vi "TestTCP.vi"() -> ()   [LabVIEW 2011]
panel:
  out "Boolean":bool
  out "Error Out":errorcluster
  out "data out":string
  in  "port":u16=9000
  in  "Stop Button":bool
  out "NaN/Path/Refnum?":bool
  in  "TCP Network Connection Refnum":refnum<k5>
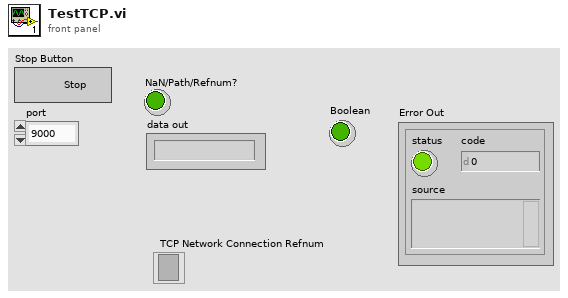
[diagram p1: front panel]
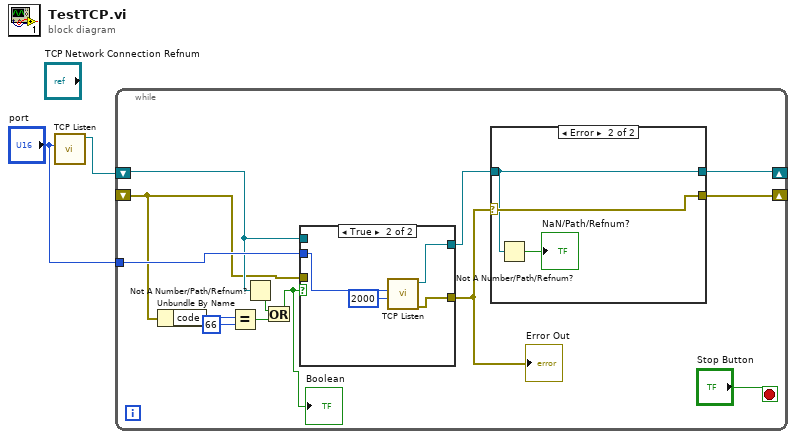
[diagram p0: block diagram]
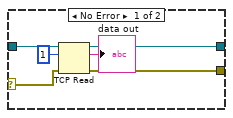
[diagram p3: hidden frame]
diagram:
  n1 = call <vilib>:"TCP Listen.vi"("port"="port") -> ("connection ID"=w2:refnum<k5>)  [unwired: 6 in, 4 out]
  n2 = while {
    shift-right: [w15] -> _
    shift-left: _ -> [w6]
    shift-right: [w14] -> _
    shift-left: w2 -> [w7]
    tunnel: "port" -> [w12]
    stop <- "Stop Button" stop-if-true
    n3 = Unbundle By Name(w6) -> ("code"=w9:i32)
    n4 = Equal?(x=w9, y=66) -> (x = y?=w10:bool)
    n5 = Not A Number/Path/Refnum?(number/path/refnum=w7) -> (NaN/Path/Refnum?=w11:bool)
    n6 = Or(x=w11, y=w10) -> (x .or. y?=w3:bool)
    "Boolean" <- w3
    n7 = case shown="True" w3 {
      tunnel: w12 -> [_ w21]
      tunnel: w7 -> [w17 _]
      tunnel: [w17 w20] -> w5
      tunnel: [w16 w19] -> w4
      tunnel: w6 -> [w16 _]
      frame False {
      }
      frame True {
        n8 = call <vilib>:"TCP Listen.vi"("timeout ms (wait forever: -1)"=2000, "port"=w21) -> ("error out"=w19:errorcluster, "connection ID"=w20:refnum<k5>)  [unwired: 5 in, 3 out]
      }
    }
    "Error Out" <- w4
    n9 = case shown="Error" w4 {
      selector: w4 -> [w25 w30]
      tunnel: w5 -> [w27 w28]
      tunnel: [w26 w30] -> w15
      tunnel: [w24 w28] -> w14
      frame No Error {
        n10 = TCP Read(connection ID=w27, bytes to read=1, error in (no error)=w25) -> (connection ID out=w24:refnum<k5>, data out=→"data out":string, error out=w26:errorcluster)  [unwired: 2 in]
      }
      frame Error {
        n11 = Not A Number/Path/Refnum?(number/path/refnum=w28) -> (NaN/Path/Refnum?=→"NaN/Path/Refnum?":bool)
      }
    }
  }
